vi "绝对标准偏差判断.vi"(9 "实测值":sgl, 10 "绝对标准偏差":dbl, 11 "标准值":dbl) -> (3 "合格？":bool)   [LabVIEW 2016, in "斯坦道总磷.lvlib"]
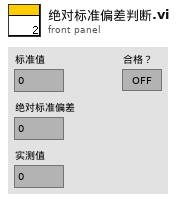
[diagram p1: front panel]
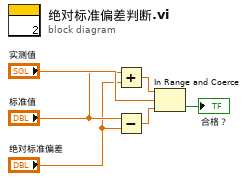
[diagram p0: block diagram]
diagram:
  n1 = Add(x="标准值", y="绝对标准偏差") -> (x+y=w2:dbl)
  n2 = Subtract(x="标准值", y="绝对标准偏差") -> (x-y=w1:dbl)
  n3 = In Range and Coerce(upper limit=w2, x="实测值", lower limit=w1) -> (In Range?=→"合格？":bool)  [unwired: 1 out]
